vi "Do Get VI Frontpanel Picture.vi"(8 "error in (no error)":errorcluster, 10 "Get VI Frontpanel Picture Argument":T3, 11 "Data Cluster in":T1) -> (0 "error out":errorcluster, 3 "Data Cluster out":T1)   [LabVIEW 2025, in "Scripting Server.lvlib"]
uses:
  Scripting Server.lvlib
  Get VI Frontpanel Picture (Reply Payload)--cluster.ctl
  Config Data.ctl
  Module Data--cluster.ctl
  Get VI Frontpanel Picture Argument--cluster.ctl
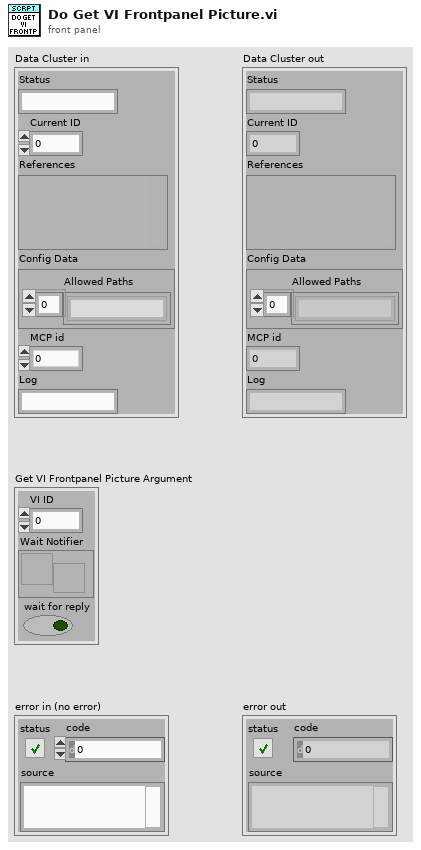
[diagram p1: front panel]
types:
  T1 = typedef "Scripting Server.lvlib/Module Data--cluster.ctl" = cluster{"Status":string, "Current ID":i32, "References":variant, "Config Data":T2, "MCP id":i32, "Log":string}
  T2 = typedef "Scripting Server.lvlib/Config Data.ctl" = cluster{"Allowed Paths":string[]}
  T3 = typedef "Scripting Server.lvlib/Get VI Frontpanel Picture Argument--cluster.ctl" = cluster{"VI ID":i32, "Wait Notifier":refnum<notifier>, "wait for reply":bool}
  T4 = typedef "Scripting Server.lvlib/Get VI Frontpanel Picture (Reply Payload)--cluster.ctl" = cluster{"VI Frontpanel Picture":picture, "error":errorcluster}
  T5 = typedef "imagedata.ctl" = cluster{"image type":i32, "image depth":i32, "image":u8[], "mask":u8[], "colors":u32[], "Rectangle":cluster{"left":i16, "top":i16, "right":i16, "bottom":i16}}
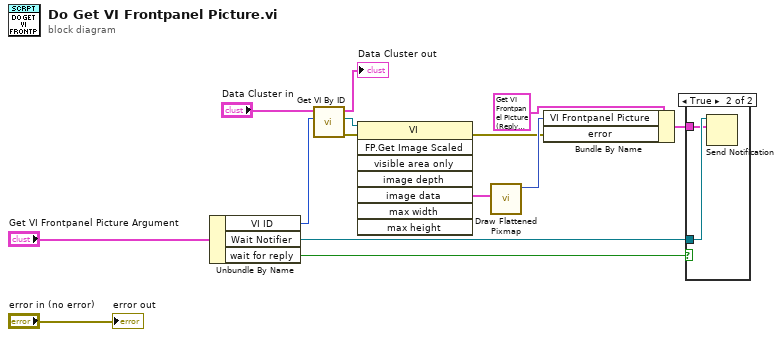
[diagram p0: block diagram]
diagram:
  n1 = Unbundle By Name("Get VI Frontpanel Picture Argument") -> ("VI ID"=w6:i32, "Wait Notifier"=w11:refnum<notifier>, "wait for reply"=w12:bool)
  n2 = call "Get VI By ID.vi"("ID"=w6, "Data Cluster in"="Data Cluster in") -> ("error out"=w5:errorcluster, "VI Reference"=w4:refnum<vi>, "Data Cluster out"=→"Data Cluster out":T1)  [unwired: 7 in]
  n3 = invoke class="VI" method="FP.Get Image Scaled"(reference=w4, error in=w5) -> (error out=w1:errorcluster, "image data"=w3:T5)  [unwired: 6 in, 6 out]
  n4 = call <vilib>:"Draw Flattened Pixmap.vi"("image data"=w3) -> ("new picture"=w2:picture)  [unwired: 8 in]
  n5 = Bundle By Name(cluster=T4 {"VI Frontpanel Picture"=bytes[0], "error"={"status"=FALSE, "code"=0, "source"=""}} ("Get VI Frontpanel Picture (Reply Payload)"), "VI Frontpanel Picture"=w2, "error"=w1) -> (w13:T4)
  n6 = case "DQMH_FIRE_NOTIFIER" shown="True" w12 {
    tunnel: w11 -> [_ w16]
    tunnel: w13 -> [_ w15]
    frame False {
    }
    frame True {
      n7 = Send Notification(notification=w15, notifier=w16) -> ()  [unwired: 1 in, 2 out]
    }
  }
  "error out" <- "error in (no error)"
